vi "Vision_Processing_L_R2.vi"(0 "Current State":enum16{"Short Range", "Long Range"}(ring)=enum."Long Range", 1 "Image Dst":T1=refnum, 2 "Inpute Image":T1=refnum, 3 "Startup Flag":bool, 4 "Valid Beacon History - in":bool[](array[boolean])=[TRUE, TRUE, TRUE, TRUE, TRUE, TRUE, TRUE, TRUE, TRUE, TRUE, TRUE, TRUE, TRUE, TRUE, TRUE, TRUE, TRUE, TRUE, TRUE, TRUE], 5 "Current ROI Descriptor":T7={"Global Rectangle"=[0, 126, 320, 179], "Contours"=[{"ID"=enum."External", "Type"=12, "Coordinates"=[0, 126, 320, 179, 0]}]} {"Contours"."Type" items=["No Selection", "Point", "Line", "Rectangle", "Oval", "Polygon", "Freehand Region", "Annulus", "Unused2", "Unused3", "Broken Line", "Freehand Line", "Rotated Rectangle"]}, 6 "Avg Score - Last":dbl=882.2747192382812, 7 "error in (no error)":errorcluster, 8 "Current Settings":T4={"Curve Parameters"={"Extraction Mode"=1, "Edge Threshold"=150, "Edge Filter Size"=0, "Min Length"=25, "Row Search Step Size"=15, "Col Search Step Size"=15, "Max Endpoint Gap"=2, "Closed"=TRUE, "Subpixel"=TRUE}, "Match Mode"={"Rotation"=TRUE, "Scale"=TRUE, "Occlusion"=TRUE, "Reserved"=FALSE, "Reserved"=FALSE, "Reserved"=FALSE}, "Range Settings"=[{"Match Constraints"=0, "Min"=-5.0, "Max"=5.0}, {"Match Constraints"=1, "Min"=77.28628845214844, "Max"=87.28628845214844}, {"Match Constraints"=2, "Min"=0.0, "Max"=25.0}], "Number of Matches"=1, "Minimum Match Score"=782.2747, "SubPixel Accuracy"=TRUE, "Adv. Geometric Match Options 2"=[{"Setup Data Item"=20, "Item Value"=0.0}, {"Setup Data Item"=22, "Item Value"=1.0}]} {"Curve Parameters"."Extraction Mode" items=["Normal", "Uniform Regions"]; "Curve Parameters"."Edge Filter Size" items=["Fine", "Normal", "Contour Tracing"]; "Curve Parameters"."Max Endpoint Gap" min=0; "Curve Parameters"."Col Search Step Size" min=1 max=255 step=1; "Curve Parameters"."Row Search Step Size" min=1 max=255 step=1; "Curve Parameters"."Min Length" min=0; "Curve Parameters"."Edge Threshold" min=1 max=350 step=1; "Range Settings"."Max" format="%.2f"; "Range Settings"."Min" format="%.2f"; "Range Settings"."Match Constraints" items=["Rotation Angle (degrees)", "Scale Factor (%)", "Occlusion (%)"]; "Adv. Geometric Match Options 2"."Setup Data Item" items=["Curve Extraction Mode", "Curve Edge Threshold", "Curve Edge Filter Size", "Min Curve Length", "Curve Row Search Step Size", "Curve Col Search Step Size", "Curve Max Endpoint Gap", "Extract Closed Curves", "Enable Subpixel Curve Extraction", "Enable Correlation Score", "Enable Subpixel Accuracy", "Subpixel Iterations", "Subpixel Tolerance", "Initial Match List Length", "Enable Target Template Curve Score", "Min Match Separation Distance", "Min Match Separation Angle", "Min Match Separation Scale", "Max Match Overlap", "Enable Coarse Result", "Enable Calibration Support", "Enable Contrast Reversal", "Search Strategy", "Refinement Match Factor", "Subpixel Match Factor"]}, 9 "Sub Beacon Search Enable":bool[](array[boolean])=[FALSE, FALSE, FALSE, FALSE, FALSE], 13 "Avg Scale - Last":dbl=82.28628845214844, 14 "Valid Score History":dbl[](array[numeric])=[882.2267456054688, 879.6480102539062, 889.1240844726562, 884.991455078125, 875.38330078125, 881.3228759765625, 879.0923461914062, 884.8130493164062, 869.0428466796875, 879.3259887695312, 878.3837280273438, 878.5771484375, 878.74462890625, 883.9327392578125, 889.0577392578125, 886.224365234375, 888.1887817382812, 886.6435546875, 888.8932495117188, 880.26025390625] format="%#_13g", 15 "Valid Scale History":dbl[](array[numeric])=[86.3126220703125, 81.15679931640625, 81.2668228149414, 81.51744842529297, 81.17774963378906, 81.44428253173828, 81.47639465332031, 81.52884674072266, 81.38125610351562, 86.32369232177734, 81.46265411376953, 81.3922348022461, 81.34772491455078, 81.08159637451172, 81.33423614501953, 81.38683319091797, 81.22872924804688, 81.17185974121094, 81.34151458740234, 81.41799926757812] format="%#_13g", 16 "History Size":i32=20) -> (10 "Valid Scale History\nOut":dbl[](array[numeric])=[81.32903289794922, 86.3126220703125, 81.15679931640625, 81.2668228149414, 81.51744842529297, 81.17774963378906, 81.44428253173828, 81.47639465332031, 81.52884674072266, 81.38125610351562, 86.32369232177734, 81.46265411376953, 81.3922348022461, 81.34772491455078, 81.08159637451172, 81.33423614501953, 81.38683319091797, 81.22872924804688, 81.17185974121094, 81.34151458740234] format="%#_13g", 11 "Avg Scale":dbl=82.31654510498046, 12 "Avg Score":dbl=881.4775024414063, 17 "Valid Score History\nOut":dbl[](array[numeric])=[871.397216796875, 882.2267456054688, 879.6480102539062, 889.1240844726562, 884.991455078125, 875.38330078125, 881.3228759765625, 879.0923461914062, 884.8130493164062, 869.0428466796875, 879.3259887695312, 878.3837280273438, 878.5771484375, 878.74462890625, 883.9327392578125, 889.0577392578125, 886.224365234375, 888.1887817382812, 886.6435546875, 888.8932495117188] format="%#_13g", 18 "Valid Beacon History\nOut":bool[](array[boolean])=[TRUE, TRUE, TRUE, TRUE, TRUE, TRUE, TRUE, TRUE, TRUE, TRUE, TRUE, TRUE, TRUE, TRUE, TRUE, TRUE, TRUE, TRUE, TRUE, TRUE], 19 "Y Coordinates":sgl[](array[numeric])=[0.0, 0.0, 153.47913, 150.49385, 148.50107], 20 "Beacons Found":bool[](array[boolean])=[FALSE, FALSE, TRUE, TRUE, TRUE], 21 "X Coordinates":sgl[](array[numeric])=[0.0, 0.0, 161.30458, 216.11124, 265.1904], 22 "Next Main ROI Descriptor":T6={"Global Rectangle"=[0, 126, 320, 176], "Contours"=[{"ID"=enum."External", "Type"=12, "Coordinates"=[0, 126, 320, 176, 0]}]} {"Contours"."Type" items=["No Selection", "Point", "Line", "Rectangle", "Oval", "Polygon", "Freehand Region", "Annulus", "Unused2", "Unused3", "Broken Line", "Freehand Line", "Rotated Rectangle"]}, 23 "Lock Status":bool=TRUE, 24 "Startup Flag - out":bool, 25 "New Settings":T4={"Curve Parameters"={"Extraction Mode"=1, "Edge Threshold"=150, "Edge Filter Size"=0, "Min Length"=25, "Row Search Step Size"=15, "Col Search Step Size"=15, "Max Endpoint Gap"=2, "Closed"=TRUE, "Subpixel"=TRUE}, "Match Mode"={"Rotation"=TRUE, "Scale"=TRUE, "Occlusion"=TRUE, "Reserved"=FALSE, "Reserved"=FALSE, "Reserved"=FALSE}, "Range Settings"=[{"Match Constraints"=0, "Min"=-5.0, "Max"=5.0}, {"Match Constraints"=1, "Min"=77.31654510498046, "Max"=87.31654510498046}, {"Match Constraints"=2, "Min"=0.0, "Max"=25.0}], "Number of Matches"=1, "Minimum Match Score"=781.4775, "SubPixel Accuracy"=TRUE, "Adv. Geometric Match Options 2"=[{"Setup Data Item"=20, "Item Value"=0.0}, {"Setup Data Item"=22, "Item Value"=1.0}]} {"Curve Parameters"."Extraction Mode" items=["Normal", "Uniform Regions"]; "Curve Parameters"."Edge Filter Size" items=["Fine", "Normal", "Contour Tracing"]; "Curve Parameters"."Max Endpoint Gap" min=0; "Curve Parameters"."Col Search Step Size" min=1 max=255 step=1; "Curve Parameters"."Row Search Step Size" min=1 max=255 step=1; "Curve Parameters"."Min Length" min=0; "Curve Parameters"."Edge Threshold" min=1 max=350 step=1; "Range Settings"."Max" format="%.2f"; "Range Settings"."Min" format="%.2f"; "Range Settings"."Match Constraints" items=["Rotation Angle (degrees)", "Scale Factor (%)", "Occlusion (%)"]}, 26 "Next State":enum16{"Short Range", "Long Range"}(ring)=enum."Long Range", 27 "Right Image 2":T1(plugin-control))   [LabVIEW 2015]
uses:
  <vilib>/vision/Image Controls.llb/IMAQ Image.ctl
  <vilib>/vision/Pattern Matching.llb/IMAQ Curve Parameters.ctl
  <vilib>/vision/Pattern Matching.llb/IMAQ Match Range Setting.ctl
panel:
  in  "Scale Decay \nFactor":dbl=0.5
  in  "Scale Decay \nFactor":dbl=5.0
  in  "Valid Treshold\nfor Lock":i16=5
  in  "Horiztonall Beacon \nCushion (pixels)":sgl=12.0
  out "New Min Score":dbl=781.4775024414063
  out "New Low Scale":dbl=77.31654510498046
  out "New high Scale":dbl=87.31654510498046
  in  "Absolute\nMinimum Score":dbl=700.0
  in  "Absolute\nMaximum Scale":dbl=300.0
  in  "Absolute\nMinimum Scale":dbl=10.0
  in  "Default No Lock\nSetting Values":T5={"Min Scale"=50.0, "Max Scale"=150.0, "Min Score"=800.0}
  in  "Score\nCushion":dbl=100.0
  in  "Scale \nCushion":dbl=5.0
  in  "LR to SR\nTransition Scale":sgl=90.0
  in  "SR to LR\nTransition Scale":sgl=90.0
  in  "Timeout \nThrehsold":i32=1000
  in  "Main ROI Decay\nper Fail (pixels)":i32=25
  in  "ROI_factor(Horiztonal) LR":sgl=5.0
  in  "ROI_factor(vertical) LR":sgl=2.5
  in  "ROI_factor(vertical) SR":sgl=2.7
  in  "ROI_factor(Horiztonal) SR":sgl=2.0
  out "Current  Score":sgl=871.3972
  out "Current  Scale":sgl=81.32903
  in  "Fail Count - In":i32
  in  "Sub Beacon Template File Path - ARRAY":path[](array[path])=[path "/home/lvuser/natinst/bin/BeaconTemplates/Sub1.png", path "/home/lvuser/natinst/bin/BeaconTemplates/Sub2.png", path "/home/lvuser/natinst/bin/BeaconTemplates/Sub3.png", path "/home/lvuser/natinst/bin/BeaconTemplates/Sub4.png", path "/home/lvuser/natinst/bin/BeaconTemplates/Sub5.png"]
  in  "Short Range Template FIle Path":path=path "/home/lvuser/natinst/bin/BeaconTemplates/SR_Main.png"
  in  "Long Range Main\nBeacon File Path":path=path "/home/lvuser/natinst/bin/BeaconTemplates/LR_Main.png"
  # "FILE PATHS"
  # "INPUTS"
  # "CONFIG"
  # "OUTPUTS"
  # "Range"
  # "Range"
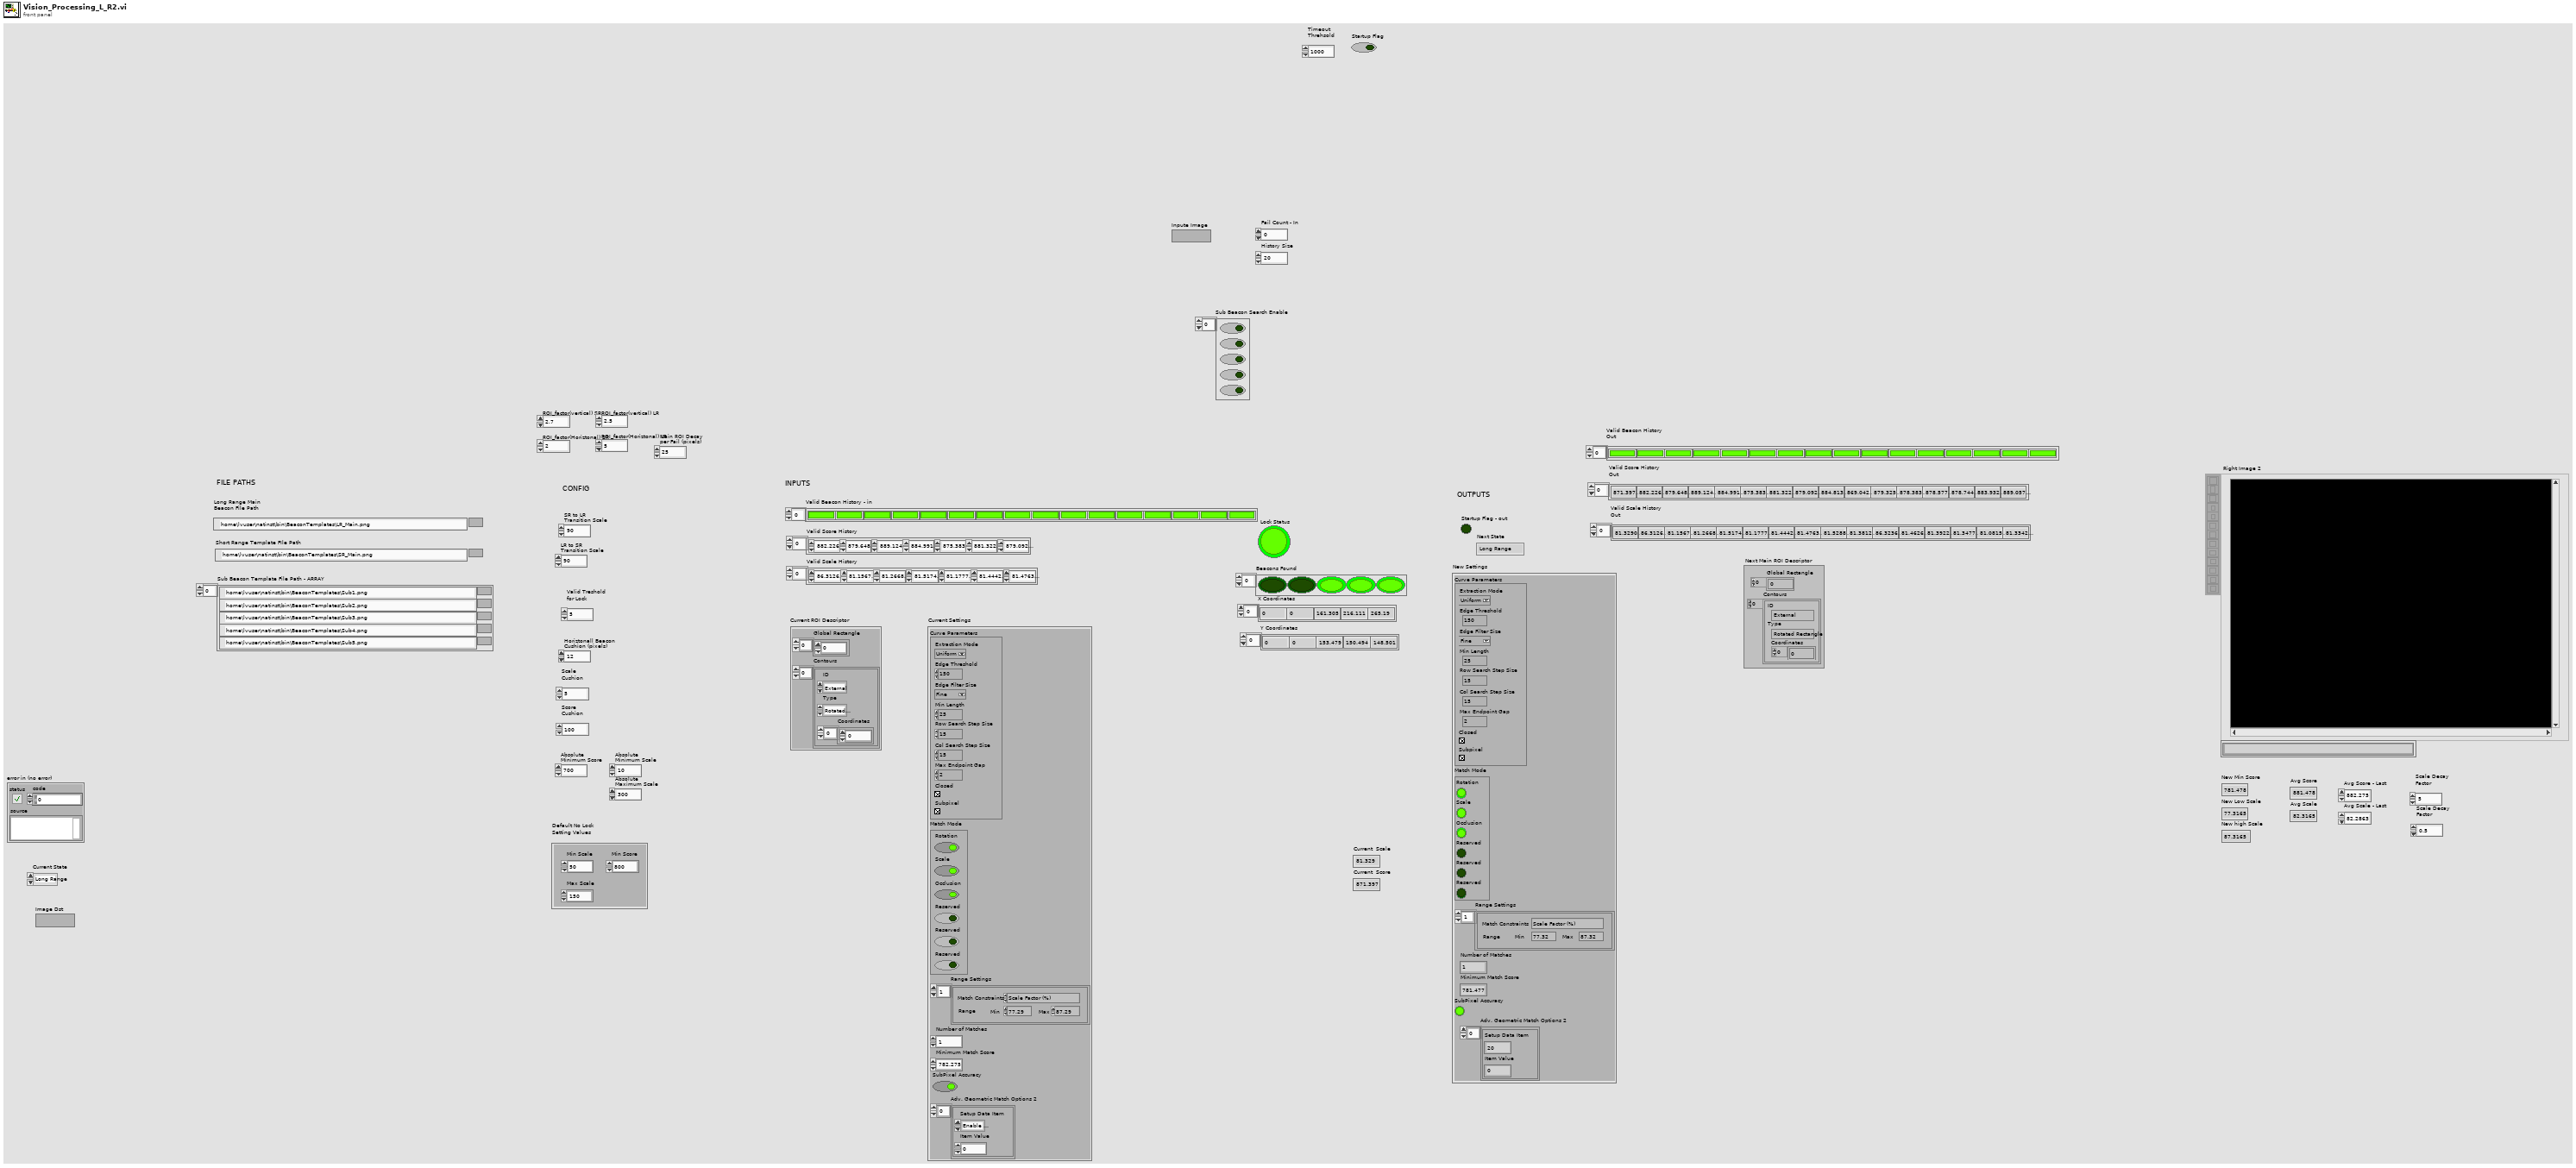
[diagram p1: front panel]
types:
  T1 = typedef "IMAQ Image.ctl" = refnum<image>
  T2 = typedef "IMAQ Curve Parameters.ctl" = cluster{"Extraction Mode":u32, "Edge Threshold":i32, "Edge Filter Size":u32, "Min Length":i32, "Row Search Step Size":i32, "Col Search Step Size":i32, "Max Endpoint Gap":i32, "Closed":bool, "Subpixel":bool}
  T3 = typedef "IMAQ Match Range Setting.ctl" = cluster{"Match Constraints":u32, "Min":dbl, "Max":dbl}
  T4 = cluster{"Curve Parameters":T2, "Match Mode":cluster{"Rotation":bool, "Scale":bool, "Occlusion":bool, "Reserved":bool, "Reserved":bool, "Reserved":bool}, "Range Settings":T3[], "Number of Matches":i32, "Minimum Match Score":sgl, "SubPixel Accuracy":bool, "Adv. Geometric Match Options 2":cluster{"Setup Data Item":u16, "Item Value":dbl}[]}
  T5 = cluster{"Min Scale":dbl, "Max Scale":dbl, "Min Score":dbl}
  T6 = typedef "ROI Descriptor" = cluster{"Global Rectangle":i32[], "Contours":cluster{"ID":enum32{"External", "Internal"}, "Type":u32, "Coordinates":i32[]}[]}
  T7 = cluster{"Global Rectangle":i32[], "Contours":cluster{"ID":enum32{"External", "Internal"}, "Type":u32, "Coordinates":i32[]}[]}
  T8 = typedef "IMAQ GM Match Report.ctl" = cluster{"Position":cluster{"x":sgl, "y":sgl}, "Angle":sgl, "Scale":sgl, "Score":sgl, "Bounding Box":cluster{"x":sgl, "y":sgl}[], "Contrast Reversed":bool, "Occlusion %":sgl, "Template Target Curve Score":sgl, "Target Template Curve Score":sgl, "Correlation Score":sgl}
  T9 = cluster{"Matches (Geometric Matching 1)[0]":T8, "Matches (Geometric Matching 1)[1]":T8, "Matches (Geometric Matching 1)[2]":T8, "Matches (Geometric Matching 1)[3]":T8, "Matches (Geometric Matching 1)[4]":T8, "Matches (Geometric Matching 1)[5]":T8, "Matches (Geometric Matching 1)[6]":T8, "Matches (Geometric Matching 1)[7]":T8, "Matches (Geometric Matching 1)[8]":T8}
  T10 = cluster{"Bounding Box[0]":cluster{"x":sgl, "y":sgl}, "Bounding Box[1]":cluster{"x":sgl, "y":sgl}, "Bounding Box[2]":cluster{"x":sgl, "y":sgl}, "Bounding Box[3]":cluster{"x":sgl, "y":sgl}, "Bounding Box[4]":cluster{"x":sgl, "y":sgl}, "Bounding Box[5]":cluster{"x":sgl, "y":sgl}, "Bounding Box[6]":cluster{"x":sgl, "y":sgl}, "Bounding Box[7]":cluster{"x":sgl, "y":sgl}, "Bounding Box[8]":cluster{"x":sgl, "y":sgl}}
  T11 = typedef "IMAQ Rectangle" = cluster{"Left":i32, "Top":i32, "Right":i32, "Bottom":i32, "Rotation":dbl}
  T12 = cluster{"index":u32, "Min Scale":dbl, "Max Scale":dbl}
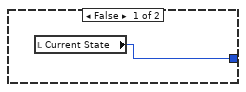
[diagram p2: hidden frame]
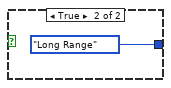
[diagram p3: hidden frame]
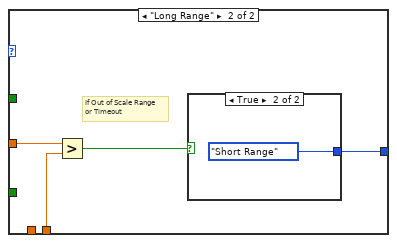
[diagram p4: hidden frame]
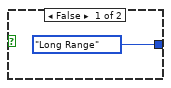
[diagram p5: hidden frame]
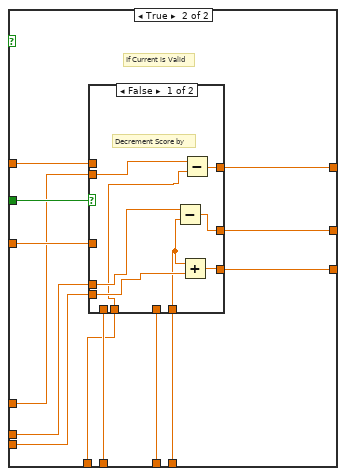
[diagram p8: hidden frame]
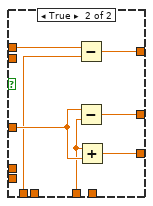
[diagram p9: hidden frame]
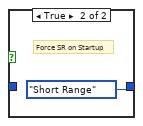
[diagram p10: hidden frame]
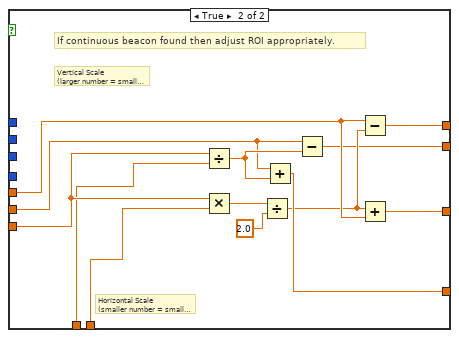
[diagram p12: hidden frame]
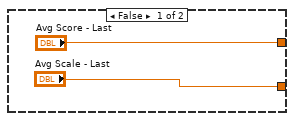
[diagram p13: hidden frame]
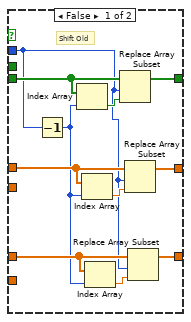
[diagram p15: hidden frame]
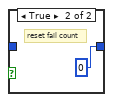
[diagram p16: hidden frame]
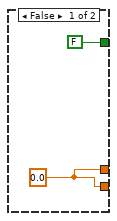
[diagram p17: hidden frame]
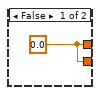
[diagram p18: hidden frame]
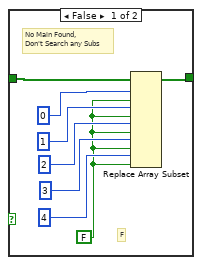
[diagram p20: hidden frame]
diagram:
  (unwired) enum16{"Short Range", "Long Range"}."Short Range"
  # "Next Settings"
  n1 = flat-sequence {
    tunnel: [w8] -> w3
    tunnel: [w7] -> w2
    tunnel: ["Image Dst"] -> w1
    tunnel: w3 -> [w139]
    tunnel: w2 -> [w137]
    tunnel: w1 -> [w138]
    frame #0 {
      # "APPLY FILTERING"
      n2 = call "Camera - Filtering"("Image In"="Inpute Image", "Image Dst"="Image Dst", "error in"="error in (no error)") -> ("Image Out"=w8:T1, "error out"=w7:errorcluster)  [unwired: 23 in]
    }
    frame #1 {
      w27 = 80.0 ("x")
      w58 = u32 1 ("index")
      w106 = u8 5
      # "Should be NEXT STATE"
      # "decay factor"
      # "Valid History"
      # "Draw ROI and stuff on outputi mage"
      # "Pull Down Startup IF Already True and Lock\nOtherwise don't update"
      # "Next Settings"
      # "Apply Limits to Settings"
      # "Scale"
      # "Min Score"
      # "Lower Scale"
      # "Upper Scale"
      # "Current Settings"
      # "Current Min\n& Max Scale"
      # "Current Valid"
      # "Update Search Settings"
      # "Next Template State"
      # "Update Template State"
      # "Calculate Average Scale/Score"
      # "Update Main ROI"
      # "Choose ROI Scale Factor"
      # "max avg"
      # "Min Required to use avarage"
      # "Valid  Ccount\n(up to 3)"
      # "****# of previous in history that must be true\nin order for position to be considered \"locked\""
      # "Update Shift Arrays"
      # "# of Beacons Found to be valid"
      # "Beacon - Y"
      # "Beacon - X"
      # "Beacons Found"
      # "Build ROI for Individual Beacons Based on Main Bounding Box"
      # "Starting X Lower Bound"
      # "Length of\nIndividual Beacon ROI"
      # "Length of Bounding Box"
      # "# of beacons"
      # "Outer Beacon Indexes"
      # "Matches"
      # "image out"
      n3 = case shown="False" "Startup Flag" {
        tunnel: [w204 enum16{"Short Range", "Long Range"}."Short Range"] -> w78
        tunnel: "Current State" -> [w204 _]
        frame False {
        }
        frame True {
          # "Force SR on Startup"
        }
      }
      n4 = case shown="\"Short Range\", Default" w78 {
        tunnel: w139 -> [w369 w404]
        tunnel: w138 -> [w368 w403]
        tunnel: "Current ROI Descriptor" -> [w366 w402]
        tunnel: "Current Settings" -> [w365 w401]
        tunnel: [1 0] -> _
        tunnel: [3 4] -> _
        tunnel: [w359 w395] -> w79
        tunnel: [w358 w394] -> w16
        tunnel: [w356 w392] -> w117
        tunnel: w137 -> [_ w391]
        tunnel: "Sub Beacon Search Enable" -> [w357 w390]
        tunnel: [sgl 3.0 ("y") sgl 5.0 ("y")] -> w127
        tunnel: [w354 w388] -> w125
        tunnel: [2 3] -> w118
        frame "Short Range", Default {
          n5 = call "Left Camera - Short Range"("Image In"=w369, "Image Dst"=w368, "ROI Descriptor (Geometric Matching 1)"=w366, "Settings (Geometric Matching 1)"=w365, "Template File Path (Geometric Matching 1)"="Short Range Template FIle Path") -> ("Image Out"=w358:T1, "Matches (Geometric Matching 1)"=w359:T8[], "Number of Matches (Geometric Matching 1)"=w360:i32, "error out"=w354:errorcluster)  [unwired: 19 in]
          n6 = Equal?(x=w360, y=1) -> (x = y?=w363:bool)
          n7 = case shown="True" w363 {
            tunnel: w357 -> [w377 w378]
            tunnel: [w370 w379] -> w356
            frame False {
              w371 = FALSE
              # "F"
              # "No Main Found,\nDon't Search any Subs"
              n8 = Replace Array Subset(array=w377, new element #1=w371, index #1=0 ("y"), new element #2=w371, index #2=1 ("y"), new element #3=w371, index #3=2 ("y"), new element #4=w371, index #4=3 ("y"), new element #5=w371, index #5=4 ("y")) -> (w370:bool[])
            }
            frame True {
              w380 = TRUE
              w381 = FALSE
              # "Search for MIDDLE Beacons"
              n9 = Replace Array Subset(array=w378, new element #1=w381, index #1=0 ("y"), new element #2=w380, index #2=1 ("y"), new element #3=w380, index #3=2 ("y"), new element #4=w380, index #4=3 ("y"), new element #5=w381, index #5=4 ("y")) -> (w379:bool[])
            }
          }
        }
        frame "Long Range" {
          n10 = call "Long Range"("Image In"=w404, "Image Dst"=w403, "ROI Descriptor (Geometric Matching 1)"=w402, "Settings (Geometric Matching 1)"=w401, "Template File Path (Geometric Matching 1)"="Long Range Main\nBeacon File Path", "error in"=w391) -> ("Image Out"=w394:T1, "Matches (Geometric Matching 1)"=w395:T8[], "Number of Matches (Geometric Matching 1)"=w397:i32, "error out"=w388:errorcluster)  [unwired: 18 in]
          n11 = Equal?(x=w397, y=1) -> (x = y?=w393:bool)
          n12 = case shown="True" w393 {
            tunnel: w390 -> [w412 w414]
            tunnel: [w405 w413] -> w392
            frame False {
              w406 = FALSE
              # "F"
              # "No Main Found,\nDon't Search any Subs"
              n13 = Replace Array Subset(array=w412, new element #1=w406, index #1=0 ("y"), new element #2=w406, index #2=1 ("y"), new element #3=w406, index #3=2 ("y"), new element #4=w406, index #4=3 ("y"), new element #5=w406, index #5=4 ("y")) -> (w405:bool[])
            }
            frame True {
              w415 = TRUE
              # "T"
              # "Search for ALL Beacons"
              n14 = Replace Array Subset(array=w414, new element #1=w415, index #1=0 ("y"), new element #2=w415, index #2=1 ("y"), new element #3=w415, index #3=2 ("y"), new element #4=w415, index #4=3 ("y"), new element #5=w415, index #5=4 ("y")) -> (w413:bool[])
            }
          }
        }
      }
      n15 = Array To Cluster(array=w79) -> (cluster=w135:T9)
      n16 = Unbundle By Name(w135) -> ("Matches (Geometric Matching 1)[0].Bounding Box"=w133:cluster{"x":sgl, "y":sgl}[], "Matches (Geometric Matching 1)[0].Scale"=w13:sgl, "Matches (Geometric Matching 1)[0].Score"=w42:sgl)
      "Current  Scale" <- w13
      "Current  Score" <- w42
      n17 = Array To Cluster(array=w133) -> (cluster=w134:T10)
      n18 = Unbundle By Name(w134) -> ("Bounding Box[0].x"=w20:sgl, "Bounding Box[0].y"=w19:sgl, "Bounding Box[2].x"=w18:sgl, "Bounding Box[2].y"=w17:sgl)
      n19 = Bundle("x"=w20, "y"=w19, "x"=w18, "y"=w17) -> (w14:cluster{"x":sgl, "y":sgl, "x":sgl, "y":sgl})  [unwired: 1 in]
      n20 = call "IMAQ Overlay Rectangle"("Rectangle"=w14, "Image"=w16) -> ("Image Out"=w15:T1)  [unwired: 8 in, 1 out]
      n21 = Subtract(x=w18, y=w20) -> (x-y=w128:sgl)
      n22 = Divide(x=w128, y=w127) -> (x/y=w130:sgl)
      n23 = Multiply(x="Horiztonall Beacon \nCushion (pixels)", y=w13) -> (x*y=w12:sgl)
      n24 = Divide(x=w12, y=sgl 100.0) -> (x/y=w9:sgl)
      n25 = Subtract(x=w19, y=w9) -> (x-y=w131:sgl)
      n26 = Add(x=w9, y=w17) -> (x+y=w132:sgl)
      n27 = for {
        N: 5 -> [_]
        tunnel: w117 -> [w348] mode=indexing
        shift-right: [w342] -> _
        shift-left: w20 -> [w347]
        tunnel: w130 -> [w346]
        tunnel: w131 -> [w339]
        tunnel: w132 -> [w338]
        tunnel: [w345] -> w124 mode=indexing
        tunnel: w9 -> [w340]
        # "Divide Bounding Box"
        # "Upper Bound of Current is\nLower Bound for Next"
        n28 = case shown="True" w348 {
          tunnel: w347 -> [w349 w350]
          tunnel: w346 -> [_ w352]
          tunnel: [w349 w351] -> w342
          tunnel: [w349 w350] -> w344
          frame False {
            # "Don't Care"
          }
          frame True {
            # "X Lower Bound"
            n29 = Add(x=w350, y=w352) -> (x+y=w351:sgl)
          }
        }
        n30 = Subtract(x=w344, y=w340) -> (x-y=w343:sgl)
        n31 = Add(x=w342, y=w340) -> (x+y=w341:sgl)
        n32 = call "Bound_RO_R_R0I.vi"("Bottom Right - Y"=w338, "Right - X"=w341, "Top Left - Y"=w339, "Top  Left - x"=w343) -> ("ROI Descriptor"=w345:T6)  [unwired: 7 in]
      }
      n33 = for {
        N: 5 -> [_]
        tunnel: w16 -> [w319]
        tunnel: w125 -> [w318]
        tunnel: w124 -> [w311] mode=indexing
        tunnel: "Sub Beacon Template File Path - ARRAY" -> [w317] mode=indexing
        tunnel: [w316] -> w122 mode=indexing
        tunnel: [w315] -> w121 mode=indexing
        tunnel: [w314] -> w107 mode=indexing
        tunnel: w117 -> [w313] mode=indexing
        tunnel: "Current Settings" -> [w312]
        shift-right: [w309] -> w21
        shift-left: w15 -> [w310]
        n34 = case shown="True" w313 {
          tunnel: w319 -> [_ w332]
          tunnel: w318 -> [_ w331]
          tunnel: w311 -> [_ w330]
          tunnel: w317 -> [_ w329]
          tunnel: [w320 w325] -> w316
          tunnel: [w320 w324] -> w315
          tunnel: [FALSE w323] -> w314
          tunnel: w312 -> [_ w322]
          frame False {
            w320 = sgl 0.0 ("x")
          }
          frame True {
            n35 = call "Sub Beacon Pattern Match"("Image In"=w332, "ROI Descriptor (Geometric Matching 1)"=w330, "Settings (Geometric Matching 1)"=w322, "Template File Path (Geometric Matching 1)"=w329, "error in"=w331) -> ("Matches (Geometric Matching 1)"=w326:T8[], "Number of Matches (Geometric Matching 1)"=w327:i32)  [unwired: 19 in, 2 out]
            n36 = Equal?(x=w327, y=1) -> (x = y?=w323:bool)
            n37 = case shown="True" w323 {
              tunnel: w326 -> [_ w336]
              tunnel: [w333 w335] -> w325
              tunnel: [w333 w334] -> w324
              frame False {
                w333 = sgl 0.0 ("x")
              }
              frame True {
                n38 = Array To Cluster(array=w336) -> (cluster=w337:T9)
                n39 = Unbundle By Name(w337) -> ("Matches (Geometric Matching 1)[0].Position.x"=w335:sgl, "Matches (Geometric Matching 1)[0].Position.y"=w334:sgl)
              }
            }
          }
        }
        n40 = call "IMAQ Overlay ROI"("ROI Descriptor"=w311, "Image"=w310) -> ("Image Out"=w309:T1)  [unwired: 8 in, 1 out]
      }
      "Beacons Found" <- w107
      "X Coordinates" <- w122
      "Y Coordinates" <- w121
      n41 = local read "Current State"() -> (w80:enum16{"Short Range", "Long Range"})
      n42 = Boolean To (0,1)(Boolean=w107) -> (0, 1=w119:i16[])
      n43 = Add Array Elements(numeric array=w119) -> (sum=w120:i16)
      n44 = Array To Cluster(array=w79) -> (cluster=w83:T9)
      n45 = Greater Or Equal?(x=w120, y=w118) -> (x >= y?=w44:bool)
      n46 = Unbundle By Name(w83) -> ("Matches (Geometric Matching 1)[0].Position.x"=w88:sgl, "Matches (Geometric Matching 1)[0].Position.y"=w89:sgl, "Matches (Geometric Matching 1)[0].Scale"=w90:sgl)
      n47 = call "IMAQ Convert ROI to Rectangle"("ROI Descriptor"="Current ROI Descriptor") -> ("Rectangle"=w82:T11)  [unwired: 8 in, 1 out]
      n48 = case shown="False" w44 {
        tunnel: "Fail Count - In" -> [w307 _]
        tunnel: [w306 u16 0] -> w75
        frame False {
          n49 = Increment(x=w307) -> (x+1=w306:i32)
        }
        frame True {
          # "reset fail count"
        }
      }
      n50 = Unbundle By Name(w82) -> ("Left"=w84:i32, "Top"=w85:i32, "Right"=w86:i32, "Bottom"=w87:i32)
      n51 = Greater?(x=w75, y="Timeout \nThrehsold") -> (0:w74:bool)
      n52 = case shown="\"Long Range\"" w80 {
        tunnel: "ROI_factor(vertical) SR" -> [w207 _]
        tunnel: "ROI_factor(Horiztonal) SR" -> [w206 _]
        tunnel: "ROI_factor(vertical) LR" -> [_ w209]
        tunnel: "ROI_factor(Horiztonal) LR" -> [_ w208]
        tunnel: [w207 w209] -> w99
        tunnel: [w206 w208] -> w100
        frame "Short Range", Default {
        }
        frame "Long Range" {
        }
      }
      n53 = case shown="False" w44 {
        tunnel: w90 -> [_ w222]
        tunnel: w88 -> [_ w229]
        tunnel: w89 -> [_ w224]
        tunnel: [w214 w230] -> w94
        tunnel: [w213 w223] -> w91
        tunnel: [w212 w228] -> w92
        tunnel: [w211 w226] -> w93
        tunnel: w84 -> [w219 _]
        tunnel: w85 -> [w218 _]
        tunnel: w86 -> [w217 _]
        tunnel: w87 -> [w216 _]
        tunnel: w99 -> [_ w221]
        tunnel: w100 -> [_ w220]
        frame False {
          w210 = 5 ("y")
          n54 = Subtract(x=w219, y="Main ROI Decay\nper Fail (pixels)") -> (x-y=w214:i32)
          n55 = Subtract(x=w218, y=w210) -> (x-y=w213:i32)
          n56 = Add(x=w217, y="Main ROI Decay\nper Fail (pixels)") -> (x+y=w212:i32)
          n57 = Add(x=w216, y=w210) -> (x+y=w211:i32)
        }
        frame True {
          # "Horizontal Scale \n(smaller number = smaller ROI)"
          # "Vertical Scale \n(larger number = smaller ROI)"
          # "If continuous beacon found then adjust ROI appropriately."
          n58 = Divide(x=w222, y=w221) -> (x/y=w227:sgl)
          n59 = Multiply(x=w222, y=w220) -> (x*y=w232:sgl)
          n60 = Divide(x=w232, y=sgl 2.0) -> (x/y=w225:sgl)
          n61 = Add(x=w224, y=w227) -> (x+y=w226:sgl)
          n62 = Subtract(x=w224, y=w227) -> (x-y=w223:sgl)
          n63 = Subtract(x=w229, y=w225) -> (x-y=w230:sgl)
          n64 = Add(x=w229, y=w225) -> (x+y=w228:sgl)
        }
      }
      n65 = Decrement(x="History Size") -> (x-1=w115:i32)
      n66 = for {
        N: "History Size" -> [_]
        shift-right: [w284] -> w35
        shift-left: "Valid Beacon History - in" -> [w272]
        tunnel: w115 -> [w280]
        shift-right: [w277] -> w48
        shift-left: "Valid Score History" -> [w279]
        shift-right: [w276] -> w47
        shift-left: "Valid Scale History" -> [w278]
        tunnel: w42 -> [w275]
        tunnel: w13 -> [w274]
        tunnel: w44 -> [w273]
        i -> [w283]
        # "Reverse Index"
        n67 = Subtract(x=w280, y=w283) -> (x-y=w281:i32)
        n68 = Equal To 0?(x=w281) -> (x = 0?=w282:bool)
        n69 = case shown="True" w282 {
          tunnel: w281 -> [w285 w304]
          tunnel: w272 -> [w295 w297]
          tunnel: [w293 w296] -> w284
          tunnel: w273 -> [_ w305]
          tunnel: w279 -> [w290 w303]
          tunnel: w278 -> [w289 w302]
          tunnel: [w288 w300] -> w277
          tunnel: [w287 w301] -> w276
          tunnel: w275 -> [_ w299]
          tunnel: w274 -> [_ w298]
          frame False {
            # "Shift Old"
            n70 = Decrement(x=w285) -> (x-1=w286:i32)
            n71 = Index Array(array=w295, index=w286) -> (element=w294:bool)
            n72 = Index Array(array=w290, index=w286) -> (element=w292:dbl)
            n73 = Index Array(array=w289, index=w286) -> (element=w291:dbl)
            n74 = Replace Array Subset(array=w295, new element=w294, index=w285) -> (w293:bool[])
            n75 = Replace Array Subset(array=w290, new element=w292, index=w285) -> (w288:dbl[])
            n76 = Replace Array Subset(array=w289, new element=w291, index=w285) -> (w287:dbl[])
          }
          frame True {
            # "Scale"
            # "Score"
            # "Valid"
            # "insert New"
            n77 = Replace Array Subset(array=w303, new element=w299, index=w304) -> (w300:dbl[])
            n78 = Replace Array Subset(array=w302, new element=w298, index=w304) -> (w301:dbl[])
            n79 = Replace Array Subset(array=w297, new element=w305, index=w304) -> (w296:bool[])
          }
        }
      }
      "Valid Beacon History\nOut" <- w35
      "Valid Score History\nOut" <- w48
      "Valid Scale History\nOut" <- w47
      n80 = call "Bound_RO_R_R0I.vi"("Bottom Right - Y"=w93, "Right - X"=w92, "Top Left - Y"=w91, "Top  Left - x"=w94) -> ("ROI Descriptor"=w49:T6)  [unwired: 7 in]
      "Next Main ROI Descriptor" <- w49
      n81 = Boolean To (0,1)(Boolean=w35) -> (0, 1=w111:i16[])
      n82 = Add Array Elements(numeric array=w111) -> (sum=w112:i16)
      n83 = Greater Or Equal?(x=w112, y="Valid Treshold\nfor Lock") -> (x >= y?=w45:bool)
      "Lock Status" <- w45
      n84 = Initialize Array(u8 0, w106) -> (w109:u8[])
      n85 = while {
        shift-right: [w255] -> w104
        shift-left: w109 -> [w257]
        tunnel: w35 -> [w263] mode=indexing
        shift-right: [w261] -> w102
        shift-left: u8 0 -> [w264]
        tunnel: "History Size" -> [w262]
        tunnel: w106 -> [w254]
        i -> [w256]
        stop <- w258 stop-if-true
        # "Grab Last 2 Valid Indexes"
        n86 = case shown="True" w263 {
          tunnel: w264 -> [w266 w268]
          tunnel: [w266 w271] -> w261
          tunnel: w257 -> [w265 w270]
          tunnel: w256 -> [_ w269]
          tunnel: [w265 w267] -> w255
          frame False {
          }
          frame True {
            # "Update Index\nto use"
            # "Increment\nValid Count"
            n87 = Replace Array Subset(array=w270, new element=w269, index=w268) -> (w267:u8[])
            n88 = Increment(x=w268) -> (x+1=w271:u8)
          }
        }
        n89 = Greater?(x=w256, y=w262) -> (0:w259:bool)
        n90 = Greater Or Equal?(x=w261, y=w254) -> (x >= y?=w260:bool)
        n91 = Or(x=w260, y=w259) -> (x .or. y?=w258:bool)
      }
      n92 = Greater?(x=w102, y=u8 2) -> (0:w103:bool)
      n93 = case shown="True" w103 {
        tunnel: w102 -> [_ w238]
        tunnel: w104 -> [_ w244]
        tunnel: w48 -> [_ w243]
        tunnel: w47 -> [_ w242]
        tunnel: ["Avg Score - Last" w236] -> w39
        tunnel: ["Avg Scale - Last" w235] -> w40
        frame False {
        }
        frame True {
          w241 = 0.0
          n94 = for {
            N: w238 -> [_]
            tunnel: w244 -> [w251] mode=indexing
            tunnel: w243 -> [w253]
            tunnel: w242 -> [w252]
            shift-right: [w249] -> w240
            shift-left: w241 -> [w247]
            shift-right: [w250] -> w239
            shift-left: w241 -> [w246]
            # "Fetch Last Valid Values"
            n95 = Index Array(array=w253, index=w251) -> (element=w248:dbl)
            n96 = Index Array(array=w252, index=w251) -> (element=w245:dbl)
            n97 = Add(x=w248, y=w247) -> (x+y=w249:dbl)
            n98 = Add(x=w245, y=w246) -> (x+y=w250:dbl)
          }
          n99 = To Double Precision Float(number=w238) -> (double precision float=w237:dbl)
          n100 = Divide(x=w240, y=w237) -> (x/y=w236:dbl)
          n101 = Divide(x=w239, y=w237) -> (x/y=w235:dbl)
        }
      }
      "Avg Score" <- w39
      "Avg Scale" <- w40
      n102 = case shown="True" w45 {
        tunnel: w74 -> [_ w146]
        tunnel: "SR to LR\nTransition Scale" -> [_ w145]
        tunnel: "LR to SR\nTransition Scale" -> [_ w144]
        tunnel: w40 -> [_ w143]
        tunnel: w45 -> [_ w142]
        tunnel: [w140 w141] -> w46
        frame False {
          n103 = local read "Current State"() -> (w140:enum16{"Short Range", "Long Range"})
        }
        frame True {
          # "Timeout"
          # "Image Lock"
          n104 = local read "Current State"() -> (w147:enum16{"Short Range", "Long Range"})
          n105 = case shown="\"Short Range\", Default" w147 {
            tunnel: w142 -> [_ _]
            tunnel: w143 -> [w151 w156]
            tunnel: w146 -> [_ _]
            tunnel: w145 -> [w150 _]
            tunnel: w144 -> [_ w155]
            tunnel: [w148 w154] -> w141
            frame "Short Range", Default {
              # "If Out of Scale Range\nor Timeout"
              n106 = Less?(x=w151, y=w150) -> (x < y?=w149:bool)
              n107 = case shown="False" w149 {
                tunnel: [enum16{"Short Range", "Long Range"}."Short Range" ("Current State") enum16{"Short Range", "Long Range"}."Long Range" ("Current State")] -> w148
                frame False {
                }
                frame True {
                }
              }
            }
            frame "Long Range" {
              # "If Out of Scale Range\nor Timeout"
              n108 = Greater?(x=w156, y=w155) -> (0:w157:bool)
              n109 = case shown="True" w157 {
                tunnel: [enum16{"Short Range", "Long Range"}."Long Range" ("Current State") enum16{"Short Range", "Long Range"}."Short Range" ("Current State")] -> w154
                frame False {
                }
                frame True {
                }
              }
            }
          }
        }
      }
      "Next State" <- w46
      n110 = Unbundle By Name("Current Settings") -> ("Minimum Match Score"=w71:sgl, "Range Settings"=w55:T3[])
      n111 = Index Array(array=w55, index=u32 1) -> (element=w70:T3)
      n112 = Unbundle(w70) -> ("Min"=w68:dbl, "Max"=w67:dbl)  [unwired: 1 out]
      n113 = case shown="False" w45 {
        tunnel: w44 -> [_ w188]
        tunnel: w39 -> [w166 w187]
        tunnel: w40 -> [w165 w186]
        tunnel: w71 -> [_ w185]
        tunnel: w68 -> [_ w184]
        tunnel: w67 -> [_ w183]
        tunnel: [w164 w182] -> w56
        tunnel: [w163 w181] -> w23
        tunnel: [w162 w180] -> w25
        tunnel: "Scale \nCushion" -> [w168 w179]
        tunnel: "Score\nCushion" -> [w167 w178]
        tunnel: "Scale Decay \nFactor" -> [_ w177]
        tunnel: "Scale Decay \nFactor" -> [_ w176]
        frame False {
          # "Apply No Lock Default for each Template"
          n114 = Unbundle By Name("Default No Lock\nSetting Values") -> ("Min Score"=w164:dbl, "Min Scale"=w163:dbl, "Max Scale"=w162:dbl)
          n115 = disable-structure shown="Disabled" {
            disable-tunnel: [w175 _] -> _
            disable-tunnel: [w174 _] -> _
            disable-tunnel: w168 -> [w173 _]
            disable-tunnel: w167 -> [w172 _]
            disable-tunnel: w166 -> [w171 _]
            disable-tunnel: w165 -> [w170 _]
            frame Disabled {
              n116 = Subtract(x=w171, y=w172) -> ()  [unwired: 1 out]
              n117 = Subtract(x=w170, y=w173) -> (x-y=w175:dbl)
              n118 = Add(x=w173, y=w170) -> (x+y=w174:dbl)
            }
            frame Enabled {
            }
          }
        }
        frame True {
          # "If Current is Valid"
          n119 = case shown="False" w188 {
            tunnel: w187 -> [_ w203]
            tunnel: [w194 w202] -> w182
            tunnel: w186 -> [_ w201]
            tunnel: [w193 w200] -> w181
            tunnel: [w192 w199] -> w180
            tunnel: w184 -> [w196 _]
            tunnel: w183 -> [w195 _]
            tunnel: w185 -> [w191 _]
            tunnel: w179 -> [_ w198]
            tunnel: w178 -> [_ w197]
            tunnel: w177 -> [w190 _]
            tunnel: w176 -> [w189 _]
            frame False {
              # "Decrement Score by"
              n120 = Subtract(x=w196, y=w189) -> (x-y=w193:dbl)
              n121 = Add(x=w189, y=w195) -> (x+y=w192:dbl)
              n122 = Subtract(x=w191, y=w190) -> (x-y=w194:dbl)
            }
            frame True {
              n123 = Subtract(x=w203, y=w197) -> (x-y=w202:dbl)
              n124 = Subtract(x=w201, y=w198) -> (x-y=w200:dbl)
              n125 = Add(x=w198, y=w201) -> (x+y=w199:dbl)
            }
          }
        }
      }
      n126 = And(x="Startup Flag", y=w45) -> (x .and. y?=w52:bool)
      n127 = case shown="True" w52 {
        tunnel: "Startup Flag" -> [w160 _]
        tunnel: [w160 FALSE] -> w51
        frame False {
        }
        frame True {
        }
      }
      "Startup Flag - out" <- w51
      n128 = Subtract(x=w25, y=w27) -> (x-y=w29:dbl)
      n129 = Add(x=w27, y=w23) -> (x+y=w30:dbl)
      n130 = Less?(x=w25, y=w23) -> (x < y?=w32:bool)
      n131 = Greater?(x=w23, y=w25) -> (0:w31:bool)
      n132 = Select(t=w30, s=w32, f=w25) -> (s? t:f=w24:dbl)
      n133 = Select(t=w29, s=w31, f=w23) -> (s? t:f=w22:dbl)
      n134 = Less?(x=w56, y="Absolute\nMinimum Score") -> (x < y?=w60:bool)
      n135 = Less?(x=w22, y="Absolute\nMinimum Scale") -> (x < y?=w63:bool)
      n136 = Greater?(x=w24, y="Absolute\nMaximum Scale") -> (0:w65:bool)
      n137 = Select(t="Absolute\nMinimum Score", s=w60, f=w56) -> (s? t:f=w62:dbl)
      "New Min Score" <- w62
      n138 = Select(t="Absolute\nMinimum Scale", s=w63, f=w22) -> (s? t:f=w26:dbl)
      "New Low Scale" <- w26
      n139 = Select(t="Absolute\nMaximum Scale", s=w65, f=w24) -> (s? t:f=w28:dbl)
      "New high Scale" <- w28
      n140 = Bundle("index"=w58, "Min Scale"=w26, "Max Scale"=w28) -> (w57:T12)  [unwired: 1 in]
      n141 = Replace Array Subset(array=w55, new element=w57, index=w58) -> (w59:T3[])
      n142 = call "IMAQ Overlay ROI"("ROI Descriptor"=w49, "Image"=w21) -> ("Image Out"=→"Right Image 2":T1)  [unwired: 8 in, 1 out]
      n143 = Bundle By Name(cluster="Current Settings", "Range Settings"=w59, "Minimum Match Score"=w62) -> (→"New Settings":T4)
    }
  }
